vi "Predekoder av LEIN stat 2.vi"(0 "Received":bool, 7 "notification":T12) -> (1 "Tool":T11, 4 "Tool analog value":dbl[](array[numeric]), 6 "Tool analog index":u16[](array[numeric]), 8 "Tool digital value":T1[](array[typedef]), 10 "Tool digital indexes":u16[](array[numeric]), 13 "Stroker Raw values":T2 {"PSU"."sys register" format="%04x"; "Tension Sub 2"."sys register" format="%04x"; "Tension Sub 1"."sys register" format="%04x"; "Solenoid"."valve status" format="%02x"; "Solenoid"."sys register" format="%04x"; "pressure 2"."sys register" format="%04x"; "pressure 1"."sys register" format="%04x"; "Controller"."High G monitoring" format="%02x"; "Controller"."NA" format="%02x"; "Controller"."GPIO values" format="%02x"; "Controller"."Relay status" format="%02x"; "Controller"."sys register" format="%04x"}, 15 "Node status array":T8[](array[typedef]))   [LabVIEW 2011]
uses:
  STAT2 data carrier type aware.ctl
  Tool/List of tools.ctl
  Status any node.ctl
  Defenitions/stat2/system status/Stat2 system error.ctl
  Defenitions/stat2/system status/Stat2 system task info.ctl
  Tool/Stroker/STroker Raw value indicator.ctl
  Controller local stat2.ctl
  pressure stat2.ctl
  solonoid stat2.ctl
  PSU stat2.ctl
  tensionsub stat2.ctl
  Measurments Handling/Status Digitalish.ctl
  Tool/Stroker/Stat def/Stroker system stat2.ctl
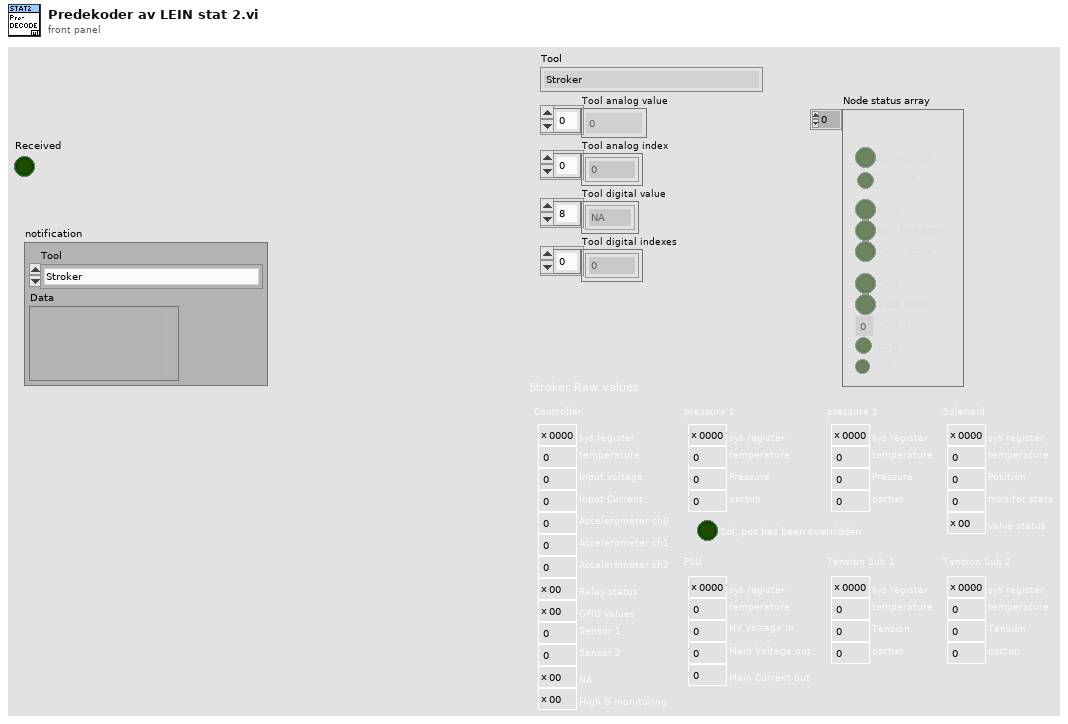
[diagram p1: front panel]
types:
  T1 = typedef "Status Digitalish.ctl" = enum16{"NA", "False", "True"}
  T2 = typedef "STroker Raw value indicator.ctl" = cluster{"Controller":T3, "pressure 1":T4, "pressure 2":T4, "Solenoid":T5, "PSU":T6, "Tension Sub 1":T7, "Tension Sub 2":T7, "Pos override used":bool}
  T3 = typedef "Controller local stat2.ctl" = cluster{"sys register":u16, "temperature":u16, "Input voltage":u16, "Input Current":u16, "Accelerometer ch0":u16, "Accelerometer ch1":u16, "Accelerometer ch2":u16, "Relay status":u8, "GPIO values":u8, "Sensor 1":i32, "Sensor 2":i32, "NA":u8, "High G monitoring":u8}
  T4 = typedef "pressure stat2.ctl" = cluster{"sys register":u16, "temperature":u16, "Pressure":u16, "osctun":u8}
  T5 = typedef "solonoid stat2.ctl" = cluster{"sys register":u16, "temperature":u16, "Position":i16, "monitor state":u8, "valve status":u8}
  T6 = typedef "PSU stat2.ctl" = cluster{"sys register":u16, "temperature":u16, "HV Voltage in":u16, "Main Voltage out":u16, "Main Current out":u16}
  T7 = typedef "tensionsub stat2.ctl" = cluster{"sys register":u16, "temperature":u16, "Tension":i16, "osctun":u8}
  T8 = typedef "Status any node.ctl" = cluster{"Name":string, "Connected":bool, "Stopped":bool, "Error":T9, "Task":T10}
  T9 = typedef "Stat2 system error.ctl" = cluster{"Error":bool, "Has had error":bool, "Com. issue":bool}
  T10 = typedef "Stat2 system task info.ctl" = cluster{"Task":bool, "Task error":bool, "Task cnt.":u8, "Job 0":bool, "User":bool}
  T11 = typedef "List of tools.ctl" = enum16{"Stroker", "Driller", "Tractor"}
  T12 = typedef "STAT2 data carrier type aware.ctl" = cluster{"Tool":T11, "Data":variant}
  T13 = typedef "Stroker system stat2.ctl" = cluster{"Controller local":T3, "pressure 1":T4, "pressure 2":T4, "solonoid":T5, "PSU":T6, "Tension Sub 1":T7, "Tension Sub 2":T7}
  T14 = typedef "Analog values for digital calculations.ctl" = cluster{"P1":dbl, "P2":dbl, "Solenoid position":dbl, "Force(bar) Inn":dbl, "Force(bar) Out":dbl, "Stroke force":dbl}
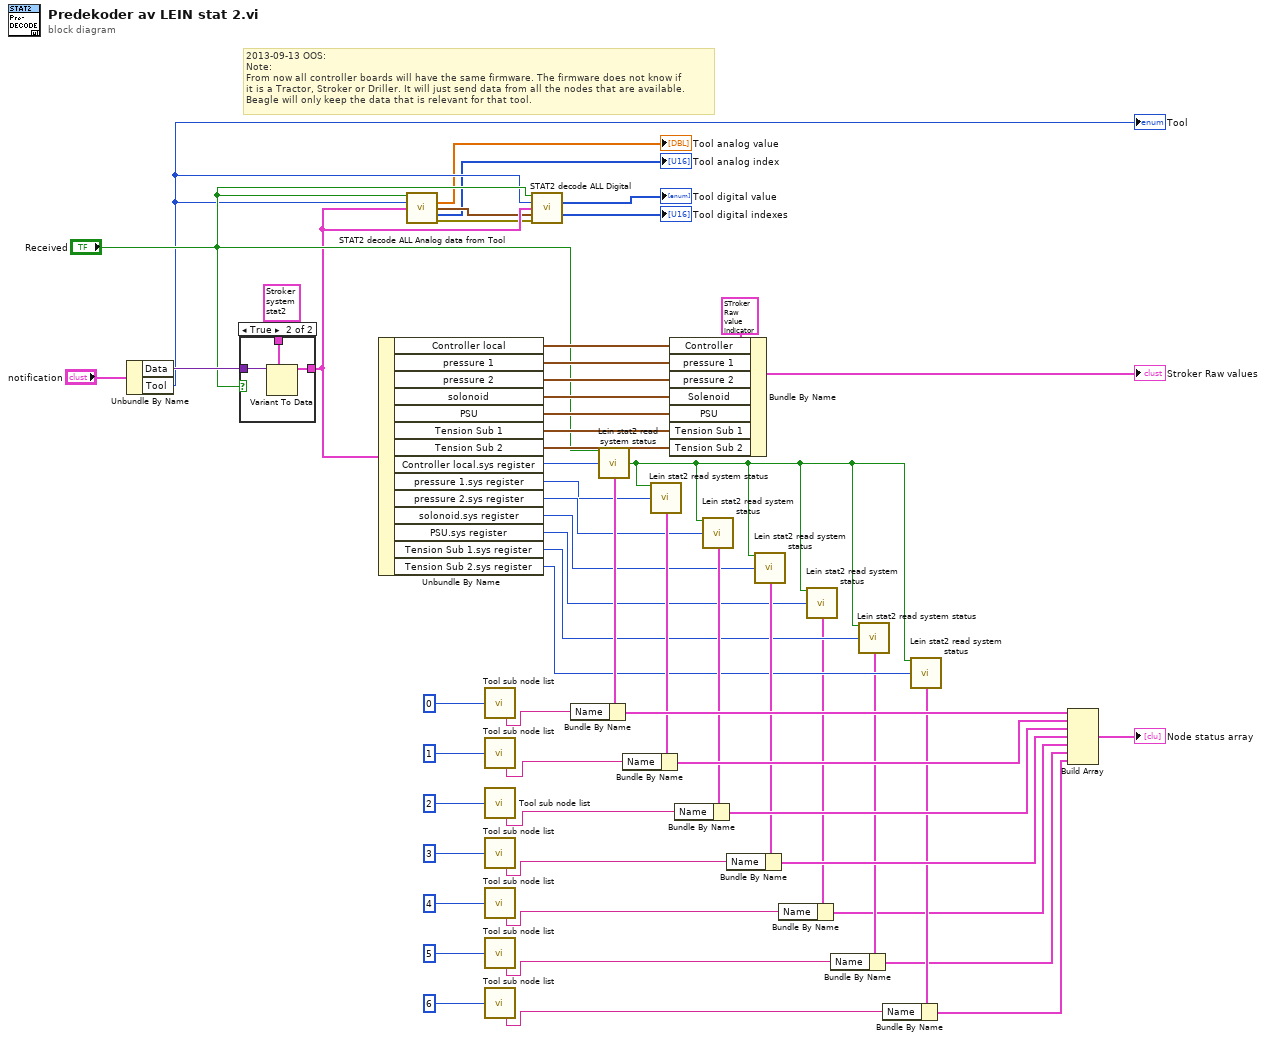
[diagram p0: block diagram]
diagram:
  # "2013-09-13 OOS:\nNote: \nFrom now all controller boards will have the same firmware. The firmware does not know if\nit is a Tractor, Stroker or Driller. It will just send data from all the nodes that are available. \nBeagle will only keep the data that is relevant for that tool."
  n1 = Unbundle By Name("notification") -> ("Data"=w56:variant, "Tool"=w8:T11)
  "Tool" <- w8
  n2 = case shown="True" "Received" {
    tunnel: T13 {"Controller local"={"sys register"=0, "temperature"=0, "Input voltage"=0, "Input Current"=0, "Accelerometer ch0"=0, "Accelerometer ch1"=0, "Accelerometer ch2"=0, "Relay status"=0, "GPIO values"=0, "Sensor 1"=0, "Sensor 2"=0, "NA"=0, "High G monitoring"=0}, "pressure 1"={"sys register"=0, "temperature"=0, "Pressure"=0, "osctun"=0}, "pressure 2"={"sys register"=0, "temperature"=0, "Pressure"=0, "osctun"=0}, "solonoid"={"sys register"=0, "temperature"=0, "Position"=0, "monitor state"=0, "valve status"=0}, "PSU"={"sys register"=0, "temperature"=0, "HV Voltage in"=0, "Main Voltage out"=0, "Main Current out"=0}, "Tension Sub 1"={"sys register"=0, "temperature"=0, "Tension"=0, "osctun"=0}, "Tension Sub 2"={"sys register"=0, "temperature"=0, "Tension"=0, "osctun"=0}} ("Controller SATT 2") -> [w59 w62]
    tunnel: [w59 w61] -> w7
    tunnel: w56 -> [_ w60]
    frame False {
    }
    frame True {
      n3 = Variant To Data(type=w62, Variant=w60) -> (data=w61:T13)  [unwired: 1 in, 1 out]
    }
  }
  n4 = Unbundle By Name(w7) -> ("Controller local"=w44:T3, "pressure 1"=w45:T4, "pressure 2"=w46:T4, "solonoid"=w47:T5, "PSU"=w28:T6, "Tension Sub 1"=w27:T7, "Tension Sub 2"=w26:T7, "Controller local.sys register"=w32:u16, "pressure 1.sys register"=w33:u16, "pressure 2.sys register"=w34:u16, "solonoid.sys register"=w35:u16, "PSU.sys register"=w24:u16, "Tension Sub 1.sys register"=w23:u16, "Tension Sub 2.sys register"=w22:u16)
  n5 = call "STAT2 decode ALL Analog data from Tool.vi"("Received(T)"="Received", "Selected Tool"=w8, "Controller SATT 2"=w7) -> ("Tool analog value"=→"Tool analog value":dbl[], "Analog for digital calc"=w6:T14, "Tool analog index"=→"Tool analog index":u16[], "error out"=w5:errorcluster)  [unwired: 9 in]
  n6 = call "Tool sub node list.vi"("Tool node"=u8 0) -> ("Node name"=w49:string)  [unwired: 7 in, 7 out]
  n7 = call "Tool sub node list.vi"("Tool node"=u8 1) -> ("Node name"=w50:string)  [unwired: 7 in, 7 out]
  n8 = call "Tool sub node list.vi"("Tool node"=u8 2) -> ("Node name"=w51:string)  [unwired: 7 in, 7 out]
  n9 = call "Tool sub node list.vi"("Tool node"=u8 3) -> ("Node name"=w29:string)  [unwired: 7 in, 7 out]
  n10 = call "Tool sub node list.vi"("Tool node"=u8 4) -> ("Node name"=w15:string)  [unwired: 7 in, 7 out]
  n11 = call "Tool sub node list.vi"("Tool node"=u8 5) -> ("Node name"=w14:string)  [unwired: 7 in, 7 out]
  n12 = call "Tool sub node list.vi"("Tool node"=u8 6) -> ("Node name"=w13:string)  [unwired: 7 in, 7 out]
  n13 = call "STAT2 decode ALL Digital.vi"("Received(T)"="Received", "Selected Tool"=w8, "Controller SATT 2"=w7, "Analog for digital calc"=w6, "error in (no error)"=w5) -> ("Tool digital value"=→"Tool digital value":T1[], "Tool digital indexes"=→"Tool digital indexes":u16[])  [unwired: 8 in, 1 out]
  n14 = call "Lein stat2 read system status.vi"("higher in hierarchy connected(T)"="Received", "sys register"=w32) -> ("Connected"=w25:bool, "All status"=w36:T8)  [unwired: 6 in, 6 out]
  n15 = Bundle By Name(cluster=w36, "Name"=w49) -> (w40:T8)
  n16 = call "Lein stat2 read system status.vi"("higher in hierarchy connected(T)"=w25, "sys register"=w33) -> ("All status"=w37:T8)  [unwired: 6 in, 7 out]
  n17 = Bundle By Name(cluster=w37, "Name"=w50) -> (w41:T8)
  n18 = Bundle By Name(cluster=T2 {"Controller"={"sys register"=0, "temperature"=0, "Input voltage"=0, "Input Current"=0, "Accelerometer ch0"=0, "Accelerometer ch1"=0, "Accelerometer ch2"=0, "Relay status"=0, "GPIO values"=0, "Sensor 1"=0, "Sensor 2"=0, "NA"=0, "High G monitoring"=0}, "pressure 1"={"sys register"=0, "temperature"=0, "Pressure"=0, "osctun"=0}, "pressure 2"={"sys register"=0, "temperature"=0, "Pressure"=0, "osctun"=0}, "Solenoid"={"sys register"=0, "temperature"=0, "Position"=0, "monitor state"=0, "valve status"=0}, "PSU"={"sys register"=0, "temperature"=0, "HV Voltage in"=0, "Main Voltage out"=0, "Main Current out"=0}, "Tension Sub 1"={"sys register"=0, "temperature"=0, "Tension"=0, "osctun"=0}, "Tension Sub 2"={"sys register"=0, "temperature"=0, "Tension"=0, "osctun"=0}, "Pos override used"=FALSE} ("Stroker Raw values"), "Controller"=w44, "pressure 1"=w45, "pressure 2"=w46, "Solenoid"=w47, "PSU"=w28, "Tension Sub 1"=w27, "Tension Sub 2"=w26) -> (→"Stroker Raw values":T2)
  n19 = call "Lein stat2 read system status.vi"("higher in hierarchy connected(T)"=w25, "sys register"=w34) -> ("All status"=w38:T8)  [unwired: 6 in, 7 out]
  n20 = Bundle By Name(cluster=w38, "Name"=w51) -> (w42:T8)
  n21 = call "Lein stat2 read system status.vi"("higher in hierarchy connected(T)"=w25, "sys register"=w35) -> ("All status"=w39:T8)  [unwired: 6 in, 7 out]
  n22 = Bundle By Name(cluster=w39, "Name"=w29) -> (w43:T8)
  n23 = call "Lein stat2 read system status.vi"("higher in hierarchy connected(T)"=w25, "sys register"=w24) -> ("All status"=w21:T8)  [unwired: 6 in, 7 out]
  n24 = Bundle By Name(cluster=w21, "Name"=w15) -> (w12:T8)
  n25 = call "Lein stat2 read system status.vi"("higher in hierarchy connected(T)"=w25, "sys register"=w23) -> ("All status"=w20:T8)  [unwired: 6 in, 7 out]
  n26 = Bundle By Name(cluster=w20, "Name"=w14) -> (w11:T8)
  n27 = call "Lein stat2 read system status.vi"("higher in hierarchy connected(T)"=w25, "sys register"=w22) -> ("All status"=w19:T8)  [unwired: 6 in, 7 out]
  n28 = Bundle By Name(cluster=w19, "Name"=w13) -> (w10:T8)
  n29 = Build Array(w40, w41, w42, w43, w12, w11, w10) -> (→"Node status array":T8[])
